vi "GetType.vi"(8 "error in (no error)":errorcluster, 11 "Set Sparse Marker Indexes [SM] Msg":refnum<class "Set Sparse Marker Indexes [SM] Msg.lvclass">) -> (0 "error out":errorcluster, 2 "Data Sample":variant, 3 "Set Sparse Marker Indexes [SM] Msg":refnum<class "Set Sparse Marker Indexes [SM] Msg.lvclass">)   [LabVIEW 2016, in "CS++Fgen.lvlib" / "Set Sparse Marker Indexes [SM] Msg.lvclass"]
doc: "This VI delivers a sample of the data type format the message expects."
uses:
  Set Sparse Marker Indexes [SM] Msg.lvclass
  Set Sparse Marker Indexes [SM] Msg.lvclass/Set Sparse Marker Indexes [SM] Msg.ctl
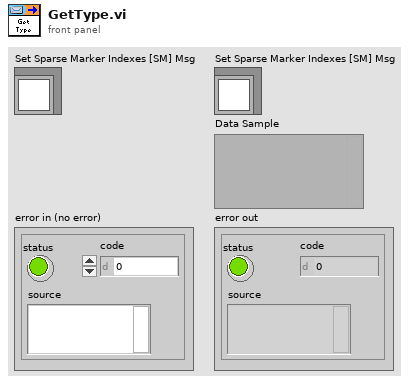
[diagram p1: front panel]
types:
  T1 = cluster{"Marker Name (\"\")":string, "Indexes Array":i64[]}
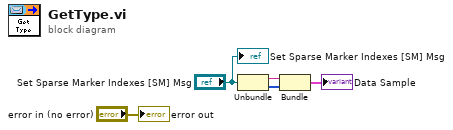
[diagram p0: block diagram]
diagram:
  n1 = Unbundle("Set Sparse Marker Indexes [SM] Msg") -> (w2:string, w1:i64[])
  n2 = Bundle("Marker Name (\"\")"=w2, "Indexes Array"=w1) -> (→"Data Sample":T1)  [unwired: 1 in]
  "error out" <- "error in (no error)"
  "Set Sparse Marker Indexes [SM] Msg" <- "Set Sparse Marker Indexes [SM] Msg"
